vi "Read Measurement.vi"(4 "Vertical Cross Value (0)":dbl, 6 "Occurrence Value (1)":i32=1, 7 "Slope Type (0: Positive)":i32(ring) items=["Positive", "Negative"], 8 "error in (no error)":errorcluster, 9 "Measurement Type (0: Frequency)":i32(ring) items=["Frequency", "Mean", "Period", "Pulse Duty", "Peak to Peak", "Cycle RMS", "Minimum", "Maximum", "Rise Time", "Fall Time", "Positive Width", "Negative Width", "Amplitude", "Cycle Mean", "High", "Low", "Negative Duty", "Positive Overshoot", "Negative Overshoot", "Cursor Mean", "Burst Width", "Positive Pulse Count", "Negative Pulse Count", "Rising Edge Count", "Falling Edge Count", "Area", "Cycle Area", "RMS", "Cursor RMS"], 10 "Channel (1: Channel 1)":i32(ring)=1 items=["Channel 1"=1, "Channel 2"=2, "Channel 3"=3, "Channel 4"=4], 11 "TDS 2000 in":refnum<class "TDS 2000.lvclass">) -> (0 "error out":errorcluster, 1 "Units":string, 2 "Measurement":dbl, 3 "TDS 2000 out":refnum<class "TDS 2000.lvclass">, 5 "Result Value":dbl)   [LabVIEW 2020, in "Oscilloscope.lvlib" / "TDS 2000.lvclass"]
uses:
  TDS 2000.lvclass
  C:/Users/ronad/Osciloscopio/Osciloscopio DQMH/Libraries/Oscilloscope/Clases/Osciloscopio/Osciloscopio.lvclass
  Osciloscopio/Osciloscopio.lvclass/Osciloscopio.ctl
  Osciloscopio/Read COM.vi
  Osciloscopio/Write COM.vi
  <instrlib>/Tektronix TDS 200 1000 2000 Series/Tektronix TDS 200 1000 2000 Series.lvlib
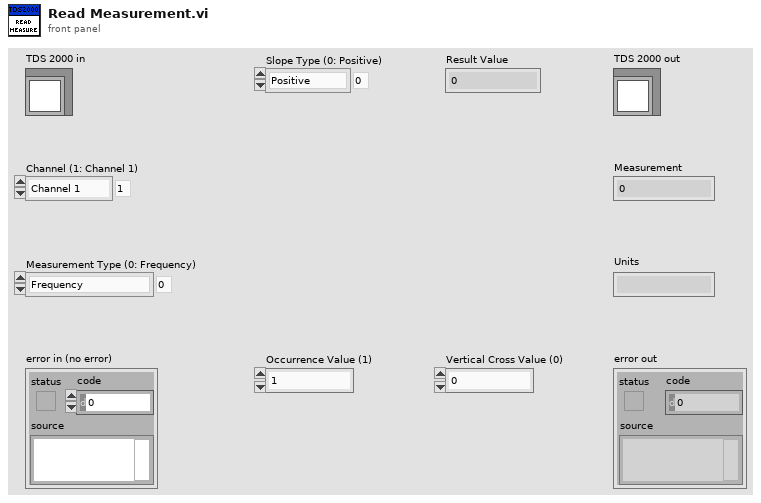
[diagram p1: front panel]
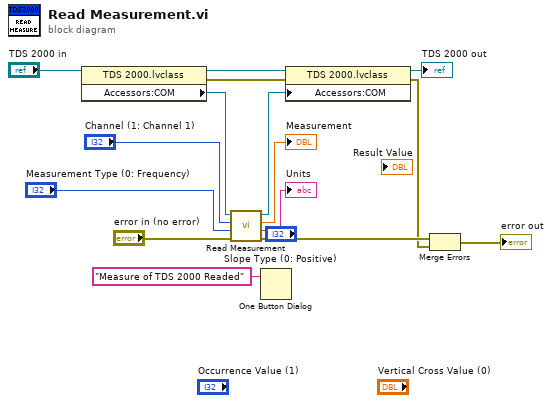
[diagram p0: block diagram]
diagram:
  n1 = property class="TDS 2000.lvclass"(reference="TDS 2000 in") -> (reference out=w12:refnum<class "TDS 2000.lvclass">, error out=w4:errorcluster, "Accessors:COM"=w14:refnum<visa-resource-name>)  [unwired: 1 in]
  n2 = call <instrlib>:"Read Measurement.vi"("error in (no error)"="error in (no error)", "Measurement Type (0: Frequency)"="Measurement Type (0: Frequency)", "Channel (1: Channel 1)"="Channel (1: Channel 1)", "VISA resource name"=w14) -> ("error out"=w7:errorcluster, "Units"=→"Units":string, "Measurement"=→"Measurement":dbl, "VISA resource name out"=w13:refnum<visa-resource-name>)  [unwired: 4 in]
  n3 = One Button Dialog(message="Measure of TDS 2000 Readed") -> ()  [unwired: 1 in, 1 out]
  n4 = property class="TDS 2000.lvclass"(reference=w12, error in=w4, "Accessors:COM"=w13) -> (reference out=→"TDS 2000 out":refnum<class "TDS 2000.lvclass">, error out=w2:errorcluster)
  n5 = Merge Errors(w7, w2) -> (→"error out":errorcluster)
